vi "GlobalGetConfigurationStatus.vi"() -> ()   [LabVIEW 2011]
panel:
  out "ConfigurationStatus":bool
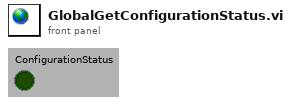
[diagram p1: front panel]
diagram:
